vi "Magazine_Set.vi"   [LabVIEW 2019]
uses:
  Magazine_Cluster.ctl
  Magazine_States.ctl
  Globals/Magazine_Globals.vi
types:
  T1 = typedef "Magazine_Cluster.ctl" = cluster{"Control_States":T2, "Magazine_Throttle":dbl, "Firing":bool}
  T2 = typedef "Magazine_States.ctl" = enum16{"No-Op", "Manual_%Vbus", "Firing", ""}
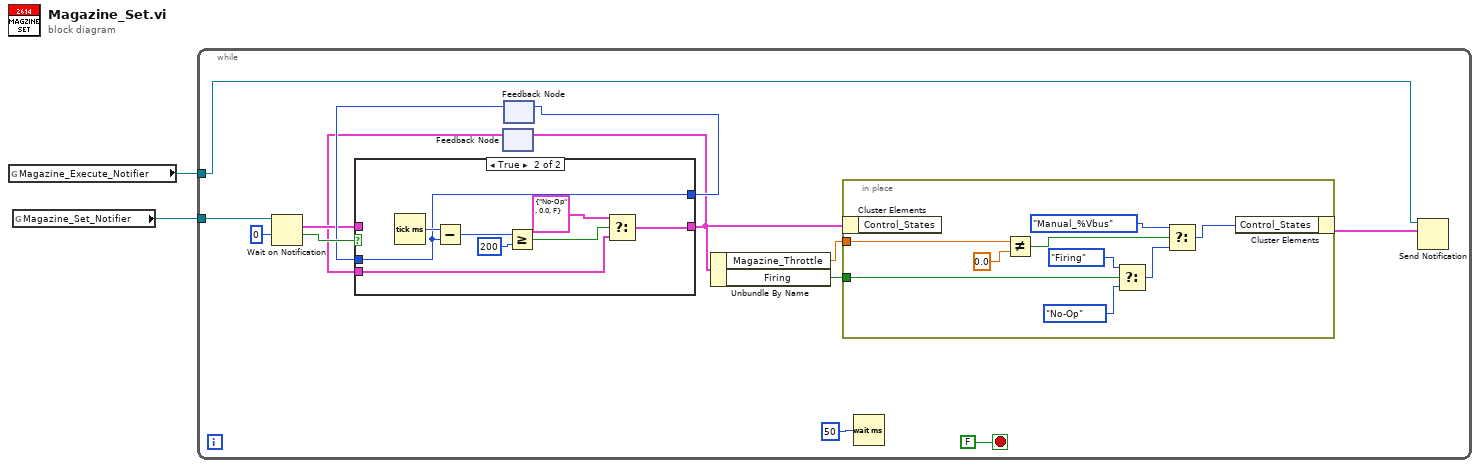
[diagram p0: block diagram]
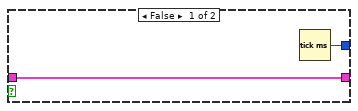
[diagram p2: hidden frame]
diagram:
  n1 = global read "Magazine_Globals.vi" "Magazine_Execute_Notifier"() -> (w2:refnum<notifier>)
  n2 = global read "Magazine_Globals.vi" "Magazine_Set_Notifier"() -> (w1:refnum<notifier>)
  n3 = while {
    tunnel: w1 -> [w5]
    tunnel: w2 -> [w3]
    stop <- FALSE stop-if-true
    n4 = Wait on Notification(notifier=w5, timeout in ms (-1)=0) -> (notification=w7:T1, timed out?=w10:bool)  [unwired: 2 in, 2 out]
    n5 = feedback #1() -> (w6:T1)  [unwired: 1 in]
    n6 = feedback #2() -> (w8:u32)  [unwired: 1 in]
    n7 = case shown="True" w10 {
      tunnel: w7 -> [w18 _]
      tunnel: [w18 w26] -> w4
      tunnel: w6 -> [_ w25]
      tunnel: [w17 w23] -> w9
      tunnel: w8 -> [_ w23]
      frame False {
        n8 = Tick Count (ms)() -> (millisecond timer value=w17:u32)
      }
      frame True {
        n9 = Tick Count (ms)() -> (millisecond timer value=w24:u32)
        n10 = Subtract(x=w24, y=w23) -> (x-y=w21:u32)
        n11 = Greater Or Equal?(x=w21, y=u32 200) -> (x >= y?=w22:bool)
        n12 = Select(t=T1 {"Control_States"=enum."No-Op", "Magazine_Throttle"=0.0, "Firing"=FALSE} ("Cluster"), s=w22, f=w25) -> (s? t:f=w26:T1)
      }
    }
    n13 = feedback-in #1(w4) -> ()
    n14 = feedback-in #2(w9) -> ()
    n15 = Unbundle By Name(w4) -> ("Magazine_Throttle"=w13:dbl, "Firing"=w12:bool)
    n16 = in-place {
      in-place-border: w13 -> [w32]
      in-place-border: w12 -> [w28]
      n17 = in-place-cluster #3(w4) -> ()  [unwired: 1 out]
      n18 = Not Equal?(x=w32, y=0.0) -> (x != y?=w27:bool)
      n19 = Select(t=Magazine_States."Firing" ("Control_States"), s=w28, f=Magazine_States."No-Op" ("Control_States")) -> (s? t:f=w31:T2)
      n20 = Select(t=Magazine_States."Manual_%Vbus", s=w27, f=w31) -> (s? t:f=w29:T2)
      n21 = in-place-cluster #3("Control_States"=w29) -> (w14:T1)
    }
    n22 = Wait (ms)(milliseconds to wait=u32 50) -> ()  [unwired: 1 out]
    n23 = Send Notification(notification=w14, notifier=w3) -> ()  [unwired: 1 in, 2 out]
  }
